vi "GENser Config Voltage Limit.vi"(7 "GEN Addr":i16=-1, 8 "error":errorcluster, 9 "Settle (0 mS)":u32, 10 "Volt Limit":dbl format="%.4f", 11 "VISA":refnum<visa-resource-name>) -> (0 "error out":errorcluster, 3 "VISA out":refnum<visa-resource-name>)   [LabVIEW 2017]
doc: "This VI sets the voltage limit (command \"PV nn\"). The power supply output will go to this limit if the load causes Constant-Voltage operation.\n\nThis VI will wait for \"Settle\" milliseconds after setting the limit to allow the output to reach the new setting. If unwired, there will be no delay\n\nNote: The voltage limit must be in the range set by the Under-Voltage Limit and the Over-Voltage Protection settings."
panel:
  # "Lambda Genesys \n Serial Port\n  DC Power Supplies"
  # "Set the Voltage Limit"
  # "-1 = no address change"
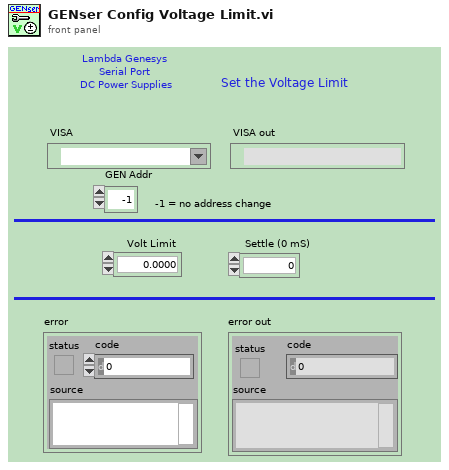
[diagram p1: front panel]
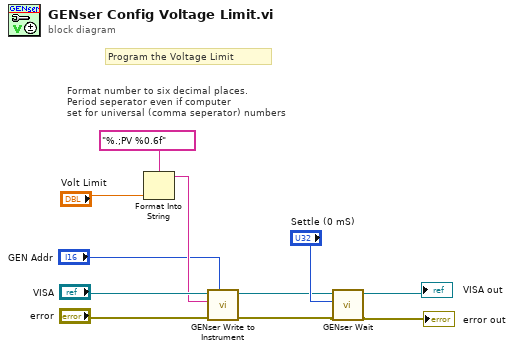
[diagram p0: block diagram]
diagram:
  # "Format number to six decimal places.\nPeriod seperator even if computer \nset for universal (comma seperator) numbers"
  # "Program the Voltage Limit"
  n1 = Format Into String(format string="%.;PV %0.6f", "Volt Limit") -> (resulting string=w4:string)  [unwired: 2 in, 1 out]
  n2 = call "GENser Write to Instrument.vi"("GEN Addr"="GEN Addr", "error"="error", "Command"=w4, "VISA"="VISA") -> ("error out"=w6:errorcluster, "VISA out"=w7:refnum<visa-resource-name>)  [unwired: 5 in, 1 out]
  n3 = call "GENser Wait.vi"("error"=w6, "Delay (20 mS)"="Settle (0 mS)", "VISA"=w7) -> ("error out"=→"error out":errorcluster, "VISA out"=→"VISA out":refnum<visa-resource-name>)  [unwired: 7 in]
